vi "Graphics-Draw Reference Lines.vi"(0 "XYGraph in":refnum<vi>, 7 "X values":dbl[](array[numeric])) -> ()   [LabVIEW 2015]
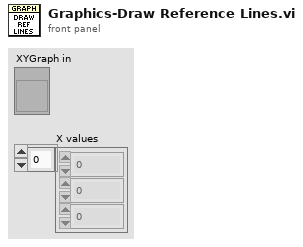
[diagram p1: front panel]
types:
  T1 = typedef "LVRectTypeDef.ctl" = cluster{"Left":i16, "Top":i16, "Right":i16, "Bottom":i16}
  T2 = cluster{"Width":u16, "Style":enum32{"Solid", "Dash", "Dot", "DashDot", "DashDotDot"}}
  T3 = typedef "LVPoint32TypeDef.ctl" = cluster{"Horizontal":i32, "Vertical":i32}
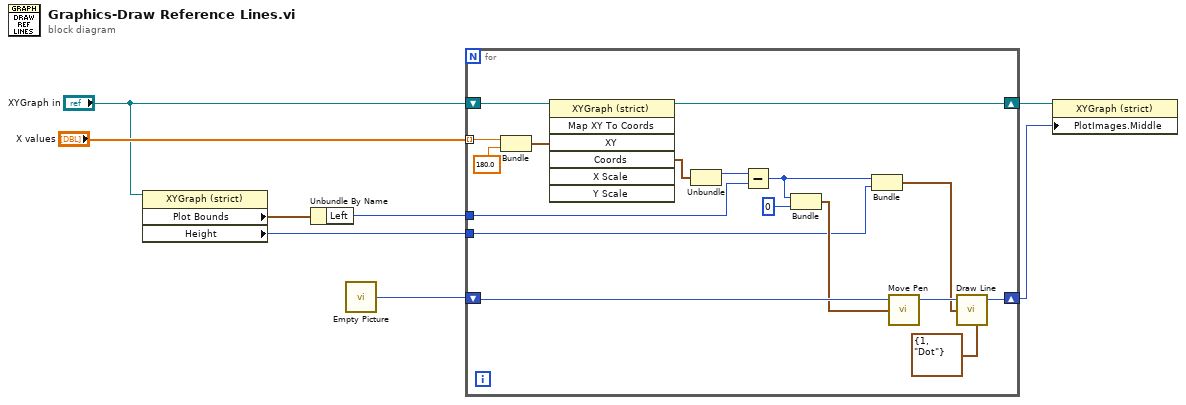
[diagram p0: block diagram]
diagram:
  n1 = property class="XYGraph (strict)"(reference="XYGraph in") -> ("Plot Bounds"=w2:T1, "Height"=w3:u32)  [unwired: 1 in, 2 out]
  n2 = Unbundle By Name(w2) -> ("Left"=w1:i16)
  n3 = call "Empty Picture"() -> ("empty picture"=w8:picture)
  n4 = for {
    tunnel: "X values" -> [w18] mode=indexing
    shift-right: [w20] -> w7
    shift-left: w8 -> [w25]
    shift-right: [w19] -> w6
    shift-left: "XYGraph in" -> [w24]
    tunnel: w1 -> [w12]
    tunnel: w3 -> [w9]
    n5 = Bundle("Numeric"=w18, 180.0) -> (w23:cluster{"Numeric":dbl, dbl})  [unwired: 1 in]
    n6 = invoke class="XYGraph (strict)" method="Map XY To Coords"(reference=w24, "XY"=w23) -> (reference out=w19:refnum<vi>, "Coords"=w17:T3)  [unwired: 5 in, 5 out]
    n7 = Unbundle(w17) -> ("Horizontal"=w16:i32)  [unwired: 1 out]
    n8 = Subtract(x=w16, y=w12) -> (x-y=w15:i32)
    n9 = Bundle(w15, 0) -> (w11:cluster{i32, i32})  [unwired: 1 in]
    n10 = Bundle(w15, "Height"=w9) -> (w14:cluster{i32, "Height":u32})  [unwired: 1 in]
    n11 = call <vilib>:"Move Pen.vi"("new position"=w11, "picture"=w25) -> ("new picture"=w21:picture)  [unwired: 3 in]
    n12 = call <vilib>:"Draw Line.vi"("picture"=w21, "end point"=w14, "pen"=T2 {"Width"=1, "Style"=enum."Dot"}) -> ("new picture"=w20:picture)  [unwired: 6 in]
  }
  n13 = property class="XYGraph (strict)"(reference=w6, "PlotImages.Middle"=w7) -> ()  [unwired: 1 in, 2 out]
